vi "main.vi"() -> ()   [LabVIEW 2024]
uses:
  TypeDefs/ModeProgram.ctl
  TypeDefs/States.ctl
  TypeDefs/producent_actions.ctl
  TypeDefs/ExtendedTimer Actions.ctl
panel:
  out "Cluster":T1={"Heater1"=FALSE, "Heater2"=FALSE, "Fan"=FALSE, "MAX_TEMP"=50.0, "TEMPERATURE"=0.0, "TIMEOUT"=0.0, "Czas_do_końca"=0.0}
  out "States":T2
  in  "Plus":bool
  out "Temperature":dbl(graph)
  out "Time":string
  in  "POWER OFF":bool
  in  "Minus":bool
  in  "Start/Stop":bool
  in  "Temperature [°C]":dbl(knob) min=0.0 max=300.0 step=1.0 scale=50.0..300.0
  in  "Mode Selector":T3 scale=0.0..3.0
  # "°C"
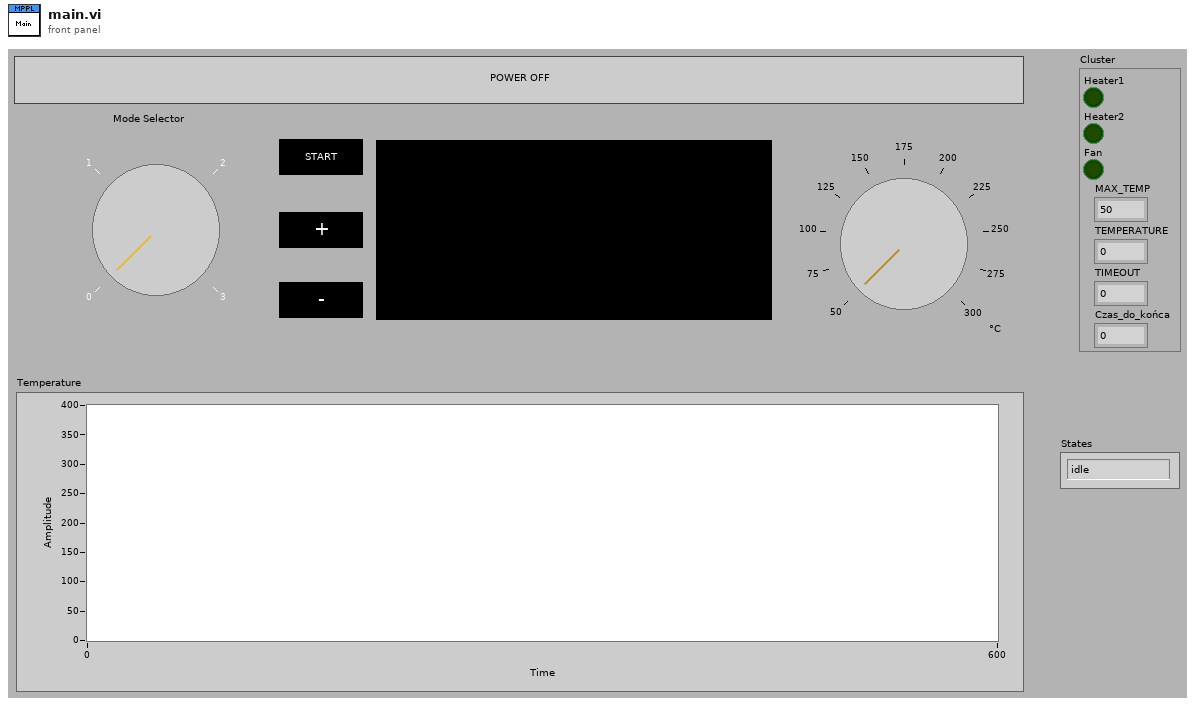
[diagram p1: front panel]
types:
  T1 = cluster{"Heater1":bool, "Heater2":bool, "Fan":bool, "MAX_TEMP":dbl, "TEMPERATURE":dbl, "TIMEOUT":dbl, "Czas_do_końca":dbl}
  T2 = typedef "States.ctl" = enum16{"idle", "reset", "heating", "stop", "exit"}
  T3 = typedef "ModeProgram.ctl" = u32
  T4 = cluster{"Heater1":bool, "Heater2":bool, "Fan":bool, "MAX_TEMP":dbl, "TEMPERATURE":dbl, "TIMEOUT":dbl, "Elapsed_Time":dbl}
  T5 = typedef "producent_actions.ctl" = enum16{"czekanie", "tryb", "temperatura", "start", "plus", "minus", "power off"}
  T6 = cluster{"Parametr":variant, "Akcje piekarnika":T5}
  T7 = typedef "ExtendedTimer Actions.ctl" = enum16{"Reset", "Check Time", "Pause", "Resume", "SetTimeOut"}
  T8 = enum8{"Enabled", "Disabled", "Disabled and Grayed Out"}
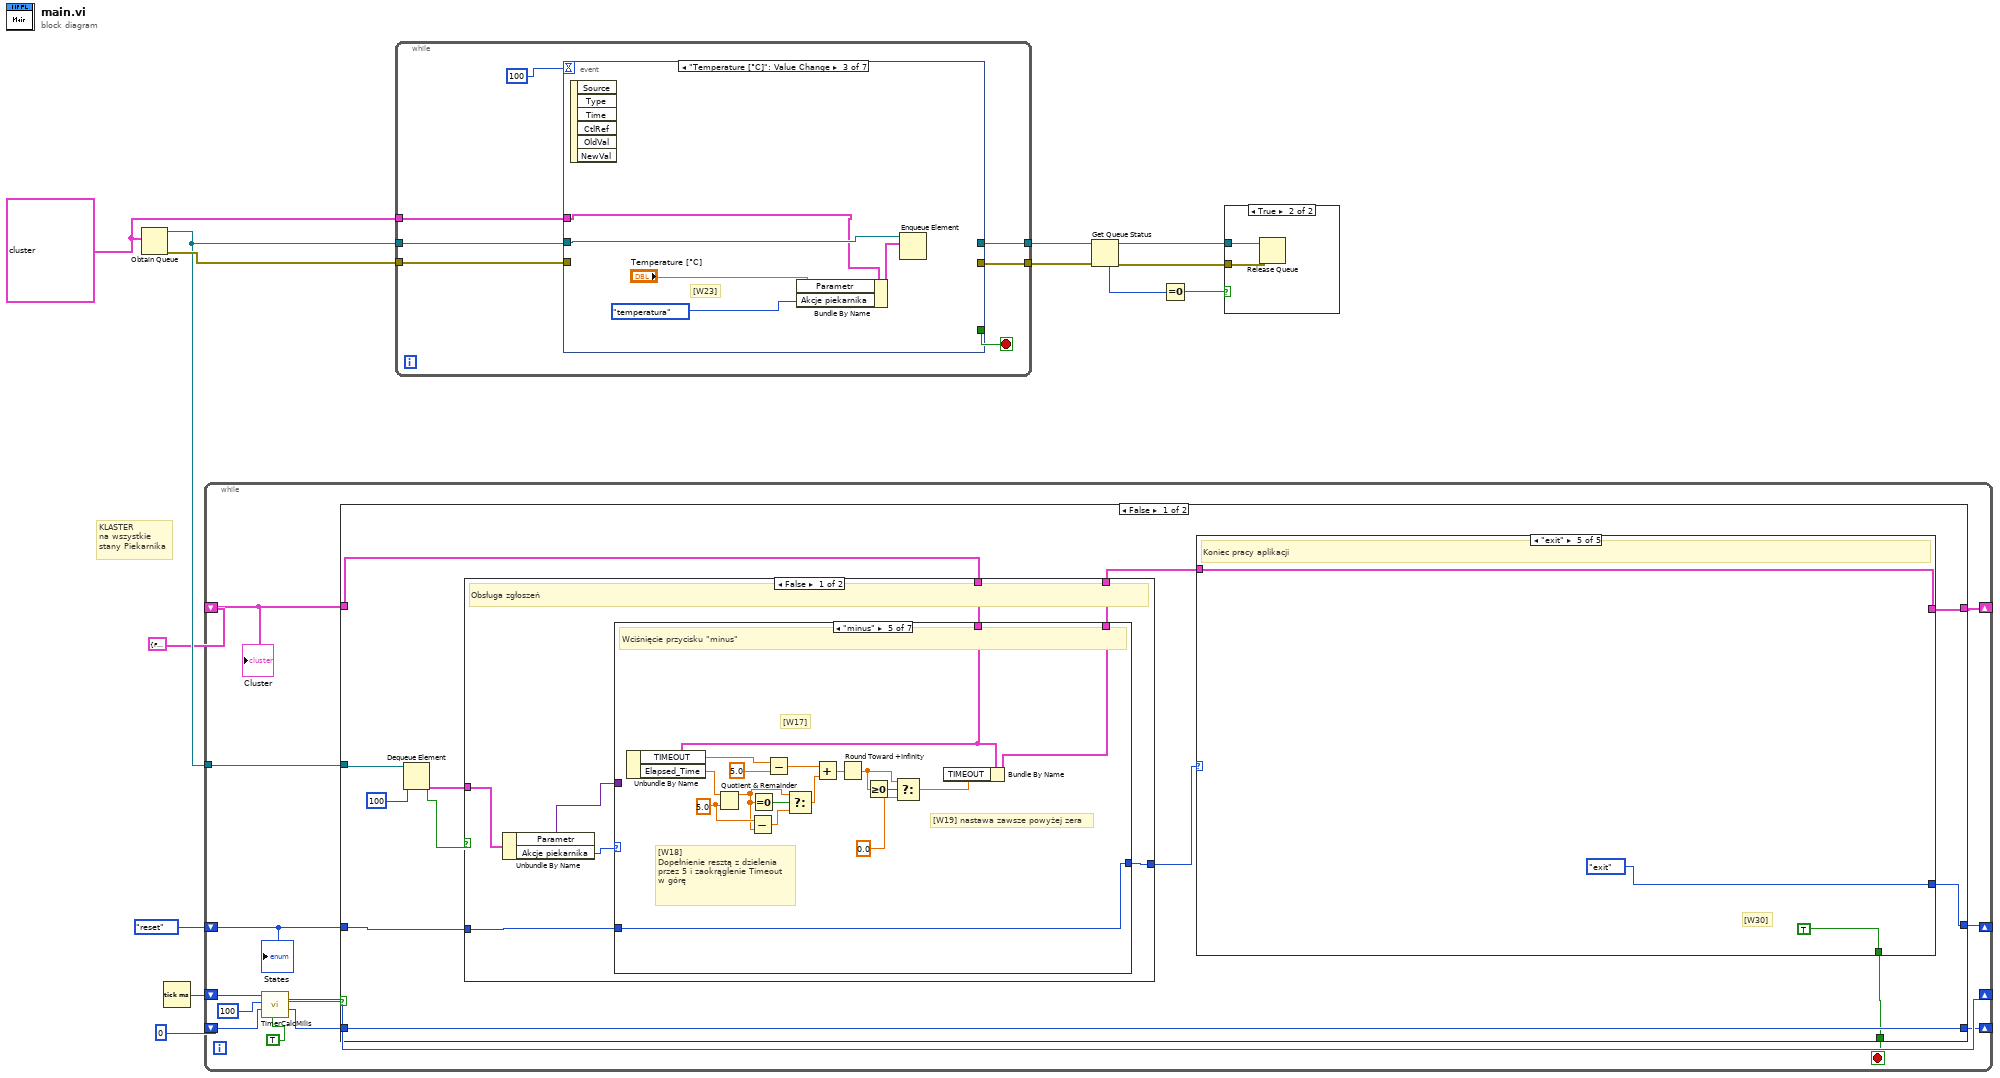
[diagram p0: block diagram]
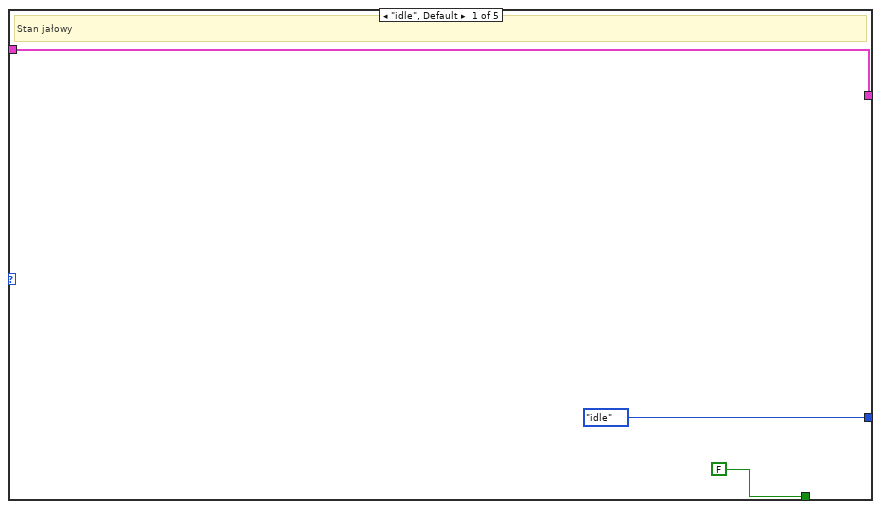
[diagram p3: hidden frame]
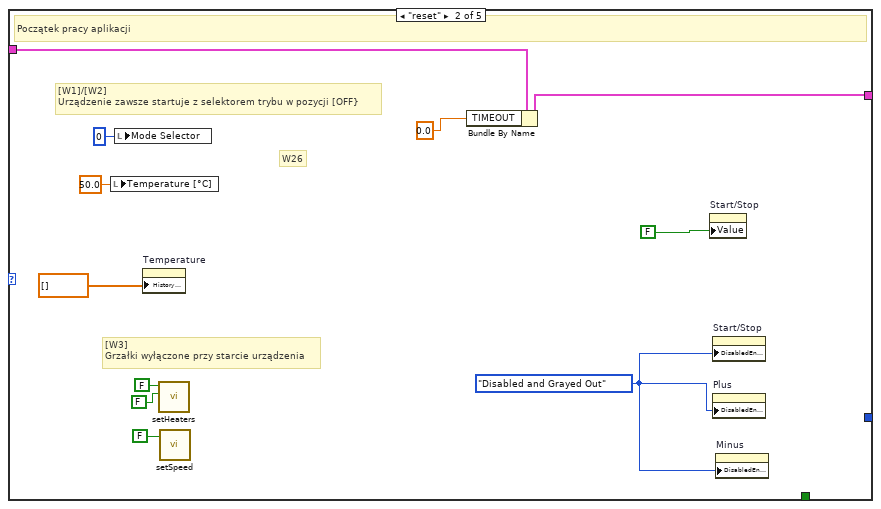
[diagram p4: hidden frame]
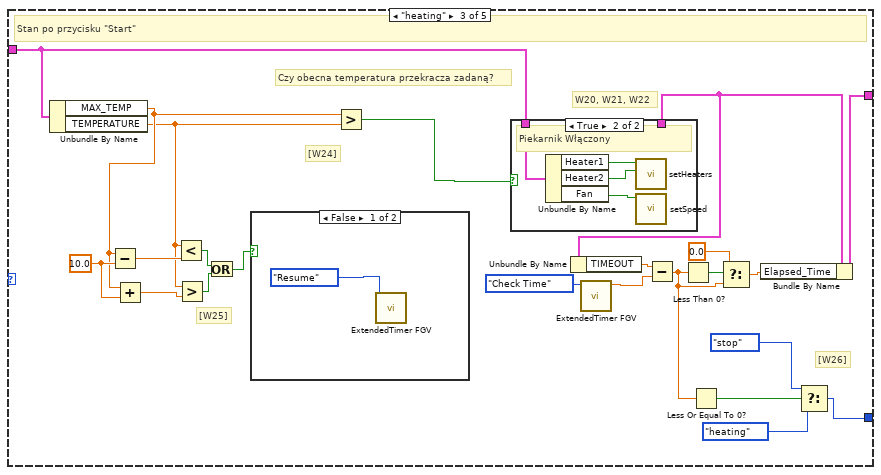
[diagram p5: hidden frame]
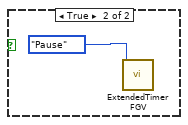
[diagram p6: hidden frame]
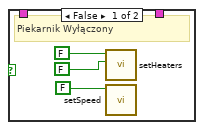
[diagram p7: hidden frame]
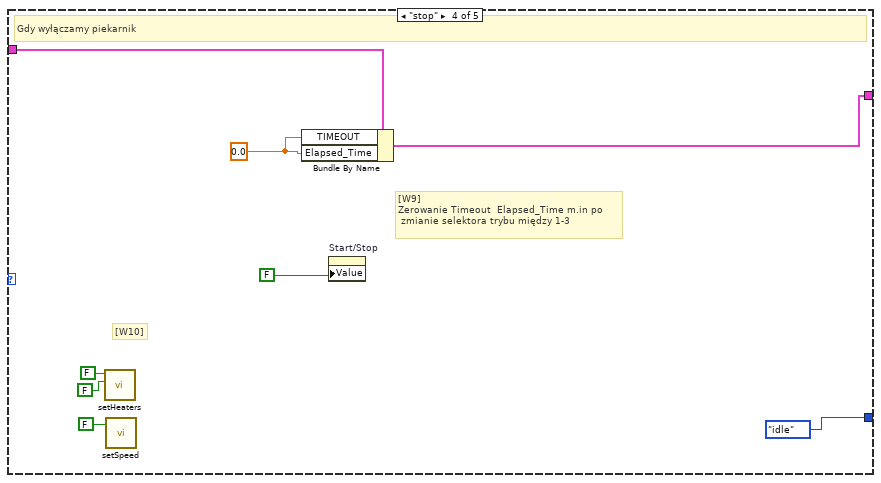
[diagram p8: hidden frame]
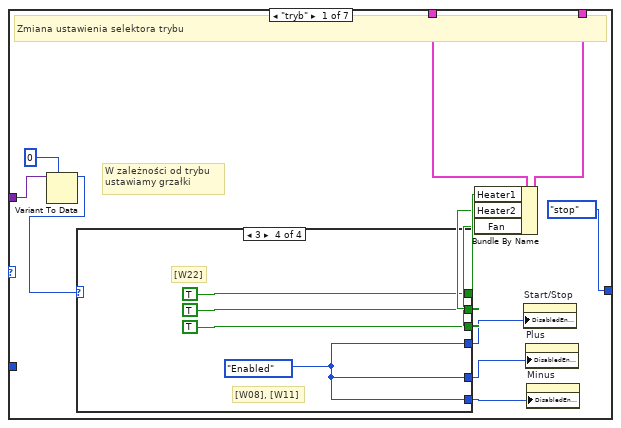
[diagram p9: hidden frame]
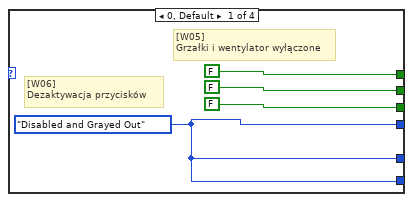
[diagram p10: hidden frame]
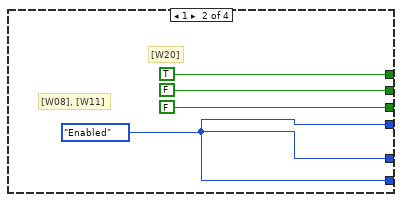
[diagram p11: hidden frame]
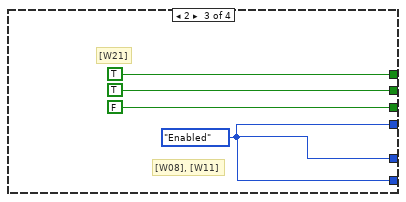
[diagram p12: hidden frame]
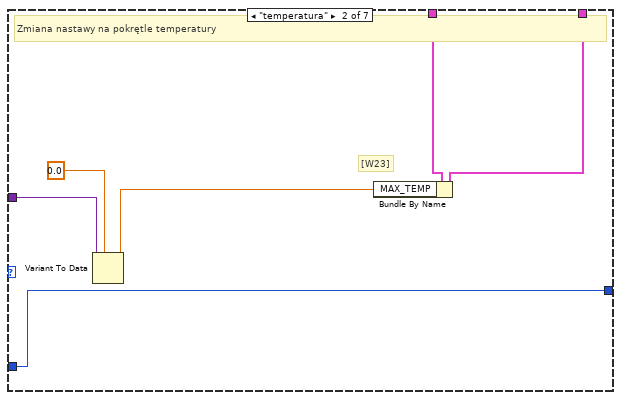
[diagram p13: hidden frame]
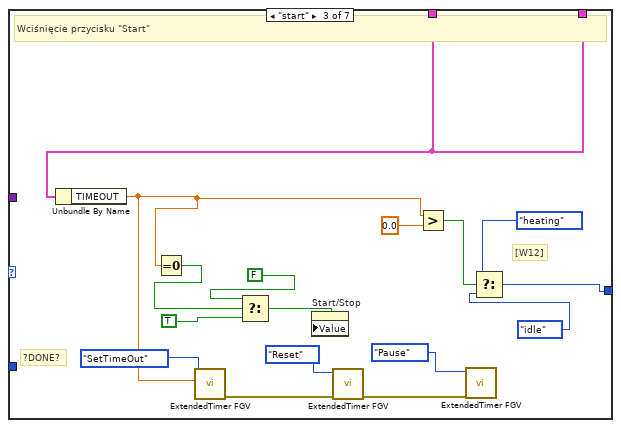
[diagram p14: hidden frame]
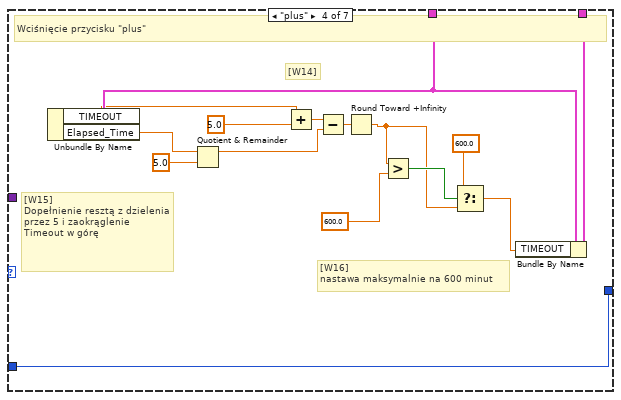
[diagram p15: hidden frame]
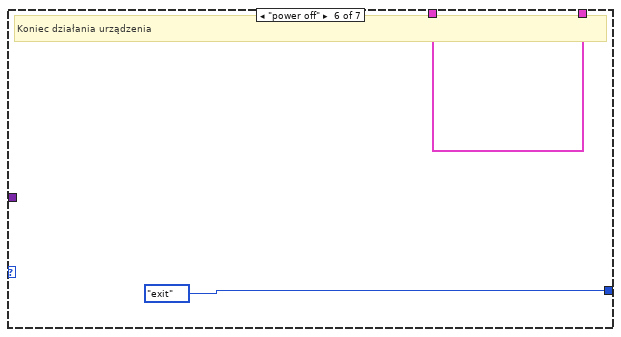
[diagram p16: hidden frame]
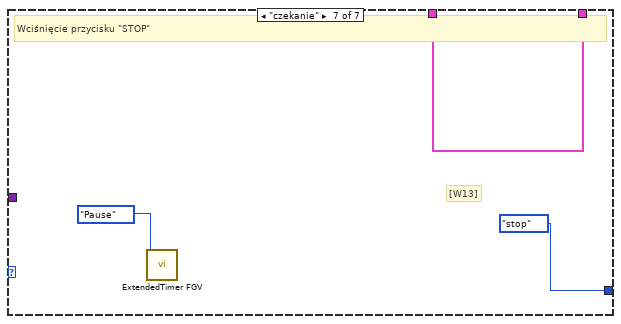
[diagram p17: hidden frame]
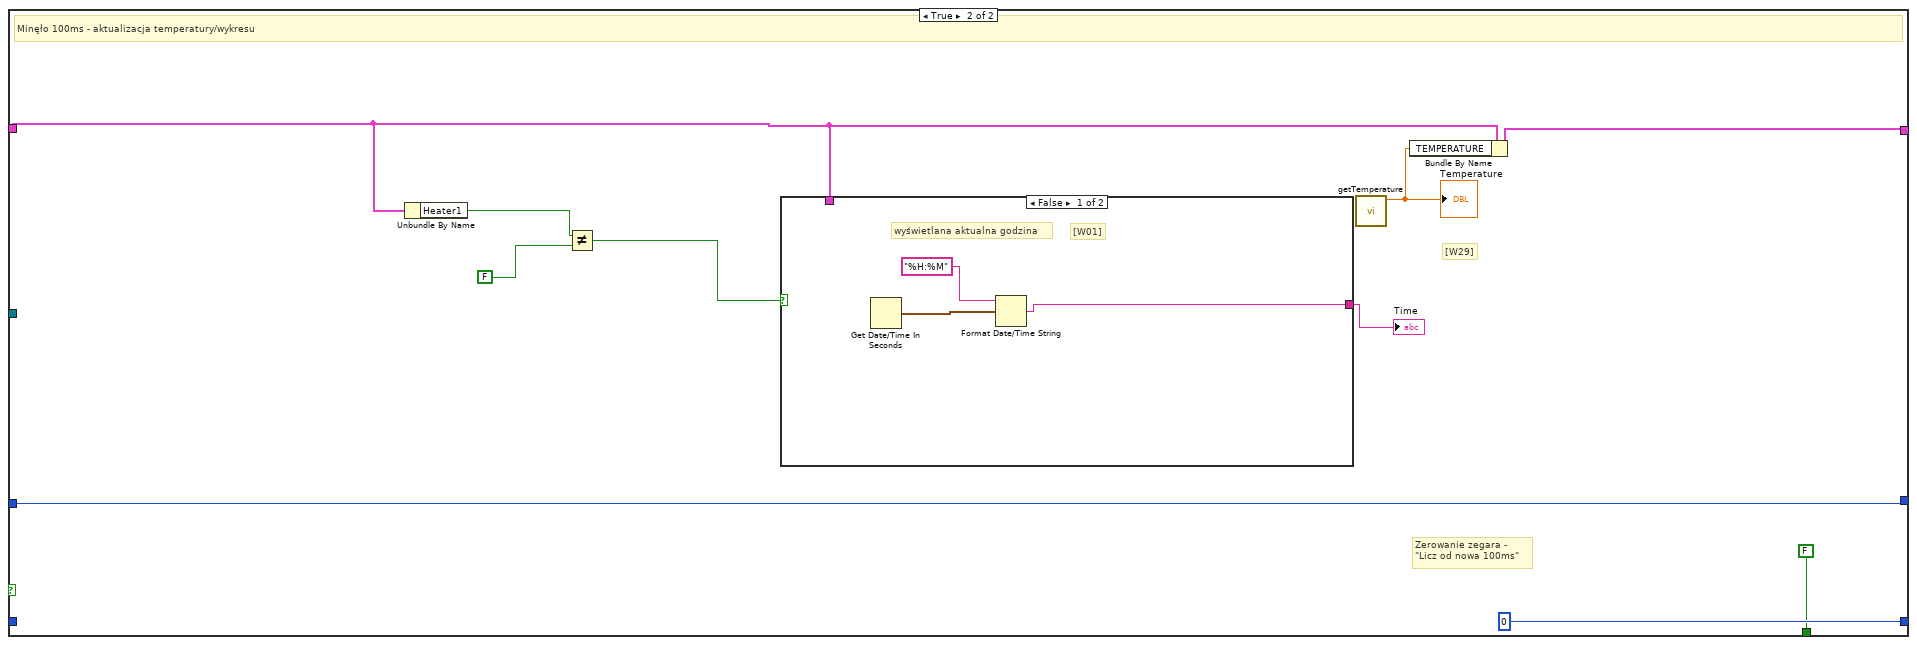
[diagram p19: hidden frame]
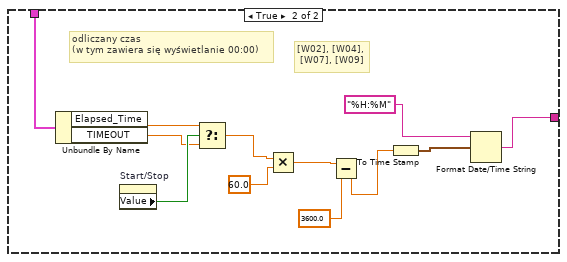
[diagram p20: hidden frame]
diagram:
  w13 = T6 {"Parametr"=variant, "Akcje piekarnika"=enum."czekanie"}
  # "KLASTER \nna wszystkie\nstany Piekarnika"
  n1 = Obtain Queue(element data type=w13) -> (queue out=w11:refnum<queue>, error out=w12:errorcluster)  [unwired: 4 in, 1 out]
  n2 = Tick Count (ms)() -> (millisecond timer value=w9:u32)
  n3 = while {
    tunnel: w11 -> [w15]
    shift-right: [w26] -> _
    shift-left: States."reset" ("States") -> [w27]
    shift-right: [w20] -> _
    shift-left: w9 -> [w23]
    shift-right: [w19] -> _
    shift-left: 0 -> [w22]
    shift-right: [w16] -> _
    shift-left: T4 {"Heater1"=FALSE, "Heater2"=FALSE, "Fan"=FALSE, "MAX_TEMP"=50.0, "TEMPERATURE"=0.0, "TIMEOUT"=0.0, "Elapsed_Time"=0.0} -> [w14]
    stop <- w17 stop-if-true
    n4 = call "TimerCalcMilis.vi"("Active"=TRUE, "ElapsedTime in"=w22, "Timeout [ms]"=u32 100, "timeOfLastCall"=w23) -> ("ElapsedTime out"=w18:u32, "Done"=w21:bool, "now"=w20:u32)  [unwired: 5 in]
    n5 = case shown="False" w21 {
      tunnel: w27 -> [w39 w199]
      tunnel: [w38 w199] -> w26
      tunnel: [w37 0] -> w19
      tunnel: w18 -> [w37 _]
      tunnel: [w36 FALSE] -> w17
      tunnel: w14 -> [w34 w198]
      tunnel: [w35 w201] -> w16
      tunnel: w15 -> [w33 _]
      frame False {
        n6 = Dequeue Element(queue=w33, timeout in ms (-1)=100) -> (element=w32:T6, timed out?=w31:bool)  [unwired: 1 in, 2 out]
        n7 = case shown="False" w31 {
          tunnel: w32 -> [w104 _]
          tunnel: w39 -> [w102 w193]
          tunnel: [w99 w193] -> w28
          tunnel: w34 -> [w101 w192]
          tunnel: [w100 w192] -> w29
          frame False {
            # "Obsługa zgłoszeń"
            n8 = Unbundle By Name(w104) -> ("Parametr"=w103:variant, "Akcje piekarnika"=w98:T5)
            n9 = case shown="\"minus\"" w98 {
              tunnel: [States."stop" ("States") w133 w148 w168 w175 States."exit" ("States") States."stop" ("States")] -> w99
              tunnel: w103 -> [w116 w138 _ _ _ _ _]
              tunnel: w102 -> [_ w133 _ w168 w175 _ _]
              tunnel: w101 -> [w105 w136 w151 w167 w185 w187 w189]
              tunnel: [w114 w135 w151 w169 w186 w187 w189] -> w100
              frame "tryb" {
                # "W zależności od trybu \nustawiamy grzałki"
                # "Zmiana ustawienia selektora trybu"
                n10 = Variant To Data(type=0, Variant=w116) -> (data=w113:i32)  [unwired: 1 in, 1 out]
                n11 = case shown="3" w113 {
                  tunnel: [FALSE TRUE TRUE TRUE] -> w112
                  tunnel: [FALSE FALSE TRUE TRUE] -> w111
                  tunnel: [FALSE FALSE FALSE TRUE] -> w110
                  tunnel: [w117 w121 w125 w129] -> w108
                  tunnel: [w117 w121 w125 w129] -> w107
                  tunnel: [w117 w121 w125 w129] -> w106
                  frame 0, Default {
                    w117 = T8."Disabled and Grayed Out" ("Disabled")
                    # "[W06]\nDezaktywacja przycisków"
                    # "[W05]\nGrzałki i wentylator wyłączone"
                  }
                  frame 1 {
                    w121 = T8."Enabled" ("Disabled")
                    # "[W20]"
                    # "[W08], [W11]"
                  }
                  frame 2 {
                    w125 = T8."Enabled" ("Disabled")
                    # "[W21]"
                    # "[W08], [W11]"
                  }
                  frame 3 {
                    w129 = T8."Enabled" ("Disabled")
                    # "[W22]"
                    # "[W08], [W11]"
                  }
                }
                n12 = Bundle By Name(cluster=w105, "Heater1"=w112, "Heater2"=w111, "Fan"=w110) -> (w114:T4)
                n13 = property on="Start/Stop" class="Bool (strict)"("DisabledEnum"=w108) -> ()  [unwired: 2 in, 2 out]
                n14 = property on="Plus" class="Bool"("DisabledEnum"=w107) -> ()  [unwired: 2 in, 2 out]
                n15 = property on="Minus" class="Bool"("DisabledEnum"=w106) -> ()  [unwired: 2 in, 2 out]
              }
              frame "temperatura" {
                # "[W23]"
                # "Zmiana nastawy na pokrętle temperatury"
                n16 = Variant To Data(type=0.0, Variant=w138) -> (data=w134:dbl)  [unwired: 1 in, 1 out]
                n17 = Bundle By Name(cluster=w136, "MAX_TEMP"=w134) -> (w135:T4)
              }
              frame "start" {
                # "[W12]"
                # "?DONE?"
                # "Wciśnięcie przycisku \"Start\""
                n18 = Unbundle By Name(w151) -> ("TIMEOUT"=w147:dbl)
                n19 = Equal To 0?(x=w147) -> (x = 0?=w146:bool)
                n20 = call "ExtendedTimer FGV.vi"("Timeout (s)"=w147, "Timer Action"=ExtendedTimer_Actions."SetTimeOut") -> ("error out"=w140:errorcluster)  [unwired: 7 in, 2 out]
                n21 = Select(t=FALSE, s=w146, f=TRUE) -> (s? t:f=w143:bool)
                n22 = property on="Start/Stop" class="Bool (strict)"("Value"=w143) -> ()  [unwired: 2 in, 2 out]
                n23 = call "ExtendedTimer FGV.vi"("error in"=w140, "Timer Action"=ExtendedTimer_Actions."Reset") -> ("error out"=w139:errorcluster)  [unwired: 7 in, 2 out]
                n24 = Greater?(x=w147, y=0.0) -> (0:w152:bool)
                n25 = call "ExtendedTimer FGV.vi"("error in"=w139, "Timer Action"=ExtendedTimer_Actions."Pause") -> ()  [unwired: 7 in, 3 out]
                n26 = Select(t=States."heating" ("States"), s=w152, f=States."idle" ("States")) -> (s? t:f=w148:T2)
              }
              frame "plus" {
                # "[W15] \nDopełnienie resztą z dzielenia przez 5 i zaokrąglenie Timeout w górę"
                # "[W16]\nnastawa maksymalnie na 600 minut"
                # "[W14]"
                # "Wciśnięcie przycisku \"plus\""
                n27 = Unbundle By Name(w167) -> ("TIMEOUT"=w166:dbl, "Elapsed_Time"=w161:dbl)
                n28 = Quotient & Remainder(x=w161, y=5.0) -> (x-y*floor(x/y)=w162:dbl)  [unwired: 1 out]
                n29 = Add(x=w166, y=5.0) -> (x+y=w164:dbl)
                n30 = Subtract(x=w164, y=w162) -> (x-y=w156:dbl)
                n31 = Round Toward +Infinity(x=w156) -> (ceil(x): smallest int >= x=w155:dbl)
                n32 = Greater?(x=w155, y=600.0) -> (0:w159:bool)
                n33 = Select(t=600.0, s=w159, f=w155) -> (s? t:f=w157:dbl)
                n34 = Bundle By Name(cluster=w167, "TIMEOUT"=w157) -> (w169:T4)
              }
              frame "minus" {
                w171 = 5.0 ("y")
                # "[W18] \nDopełnienie resztą z dzielenia przez 5 i zaokrąglenie Timeout w górę"
                # "[W17]"
                # "[W19] nastawa zawsze powyżej zera"
                # "Wciśnięcie przycisku \"minus\""
                n35 = Unbundle By Name(w185) -> ("TIMEOUT"=w183:dbl, "Elapsed_Time"=w182:dbl)
                n36 = Quotient & Remainder(x=w182, y=w171) -> (x-y*floor(x/y)=w170:dbl)  [unwired: 1 out]
                n37 = Subtract(x=w171, y=w170) -> (x-y=w172:dbl)
                n38 = Equal To 0?(x=w170) -> (x = 0?=w173:bool)
                n39 = Subtract(x=w183, y=5.0) -> (x-y=w184:dbl)
                n40 = Select(t=w170, s=w173, f=w172) -> (s? t:f=w174:dbl)
                n41 = Add(x=w184, y=w174) -> (x+y=w177:dbl)
                n42 = Round Toward +Infinity(x=w177) -> (ceil(x): smallest int >= x=w176:dbl)
                n43 = Greater Or Equal To 0?(x=w176) -> (x >= 0?=w181:bool)
                n44 = Select(t=w176, s=w181, f=0.0) -> (s? t:f=w179:dbl)
                n45 = Bundle By Name(cluster=w185, "TIMEOUT"=w179) -> (w186:T4)
              }
              frame "power off" {
                # "Koniec działania urządzenia"
              }
              frame "czekanie" {
                # "[W13]"
                # "Wciśnięcie przycisku \"STOP\""
                n46 = call "ExtendedTimer FGV.vi"("Timer Action"=ExtendedTimer_Actions."Pause") -> ()  [unwired: 8 in, 3 out]
              }
            }
          }
          frame True {
            # "Przy IDLE/Heating wystarczy\nPuścić dalej zapętlony stan\nz poprzedniej iteracji"
            # "Brak zgłoszeń/ lub błąd  = IDLE lub inny z poprzedniej iteracji"
          }
        }
        n47 = case shown="\"exit\"" w28 {
          tunnel: [States."idle" ("States") _ w70 States."idle" ("States") States."exit" ("States")] -> w38
          tunnel: [FALSE _ _ _ TRUE] -> w36
          tunnel: [w40 w49 w75 w89 w95] -> w35
          tunnel: w29 -> [w40 w50 w76 w91 w95]
          frame "idle", Default {
            # "Stan jałowy"
          }
          frame "reset" {
            w45 = T8."Disabled and Grayed Out" ("Disabled")
            # "[W3]\nGrzałki wyłączone przy starcie urządzenia"
            # "[W1]/[W2]\nUrządzenie zawsze startuje z selektorem trybu w pozycji [OFF}"
            # "W26"
            # "Początek pracy aplikacji"
            n48 = local write "Temperature [°C]"(50.0 ("Temperature [°C]")) -> ()
            n49 = local write "Mode Selector"(T3 0 ("Mode Selector")) -> ()
            n50 = property on="Temperature" class="WFChart (strict)"("History Data"=dbl[] []) -> ()  [unwired: 2 in, 2 out]
            n51 = call "setHeaters.vi"("Heater2"=FALSE ("Heater1"), "Heater1"=FALSE) -> ()  [unwired: 9 in, 1 out]
            n52 = call "setSpeed.vi"("Speed"=FALSE ("Heater1")) -> ()  [unwired: 10 in, 1 out]
            n53 = Bundle By Name(cluster=w50, "TIMEOUT"=0.0) -> (w49:T4)
            n54 = property on="Start/Stop" class="Bool (strict)"("Value"=FALSE) -> ()  [unwired: 2 in, 2 out]
            n55 = property on="Start/Stop" class="Bool (strict)"("DisabledEnum"=w45) -> ()  [unwired: 2 in, 2 out]
            n56 = property on="Plus" class="Bool"("DisabledEnum"=w45) -> ()  [unwired: 2 in, 2 out]
            n57 = property on="Minus" class="Bool"("DisabledEnum"=w45) -> ()  [unwired: 2 in, 2 out]
          }
          frame "heating" {
            w60 = 10.0 ("y")
            # "[W25]"
            # "[W26]"
            # "[W24]"
            # "W20, W21, W22"
            # "Czy obecna temperatura przekracza zadaną?"
            # "Stan po przycisku \"Start\""
            n58 = Unbundle By Name(w76) -> ("MAX_TEMP"=w59:dbl, "TEMPERATURE"=w58:dbl)
            n59 = Subtract(x=w59, y=w60) -> (x-y=w68:dbl)
            n60 = Add(x=w59, y=w60) -> (x+y=w57:dbl)
            n61 = Less?(x=w58, y=w68) -> (x < y?=w56:bool)
            n62 = Greater?(x=w58, y=w57) -> (0:w55:bool)
            n63 = Or(x=w56, y=w55) -> (x .or. y?=w54:bool)
            n64 = case shown="False" w54 {
              frame False {
                n65 = call "ExtendedTimer FGV.vi"("Timer Action"=ExtendedTimer_Actions."Resume") -> ()  [unwired: 8 in, 3 out]
              }
              frame True {
                n66 = call "ExtendedTimer FGV.vi"("Timer Action"=ExtendedTimer_Actions."Pause") -> ()  [unwired: 8 in, 3 out]
              }
            }
            n67 = Greater?(x=w59, y=w58) -> (0:w65:bool)
            n68 = case shown="True" w65 {
              tunnel: w76 -> [w82 w86]
              tunnel: [w82 w86] -> w74
              frame False {
                # "Piekarnik Wyłączony"
                n69 = call "setHeaters.vi"("Heater2"=FALSE, "Heater1"=FALSE) -> ()  [unwired: 9 in, 1 out]
                n70 = call "setSpeed.vi"("Speed"=FALSE) -> ()  [unwired: 10 in, 1 out]
              }
              frame True {
                # "Piekarnik Włączony"
                n71 = Unbundle By Name(w86) -> ("Heater1"=w85:bool, "Heater2"=w84:bool, "Fan"=w83:bool)
                n72 = call "setHeaters.vi"("Heater2"=w84, "Heater1"=w85) -> ()  [unwired: 9 in, 1 out]
                n73 = call "setSpeed.vi"("Speed"=w83) -> ()  [unwired: 10 in, 1 out]
              }
            }
            n74 = Unbundle By Name(w74) -> ("TIMEOUT"=w73:dbl)
            n75 = call "ExtendedTimer FGV.vi"("Timer Action"=ExtendedTimer_Actions."Check Time") -> ("Elapsed Time"=w67:dbl)  [unwired: 8 in, 2 out]
            n76 = Subtract(x=w73, y=w67) -> (x-y=w63:dbl)
            n77 = Less Than 0?(x=w63) -> (x < 0?=w64:bool)
            n78 = Less Or Equal To 0?(x=w63) -> (x <= 0?=w66:bool)
            n79 = Select(t=0.0, s=w64, f=w63) -> (s? t:f=w61:dbl)
            n80 = Bundle By Name(cluster=w74, "Elapsed_Time"=w61) -> (w75:T4)
            n81 = Select(t=States."stop" ("States"), s=w66, f=States."heating" ("States")) -> (s? t:f=w70:T2)
          }
          frame "stop" {
            w90 = 0.0
            # "[W9] \nZerowanie Timeout  Elapsed_Time m.in po \n zmianie selektora trybu między 1-3"
            # "[W10]"
            # "Gdy wyłączamy piekarnik"
            n82 = call "setHeaters.vi"("Heater2"=FALSE ("Heater1"), "Heater1"=FALSE) -> ()  [unwired: 9 in, 1 out]
            n83 = call "setSpeed.vi"("Speed"=FALSE ("Heater1")) -> ()  [unwired: 10 in, 1 out]
            n84 = Bundle By Name(cluster=w91, "TIMEOUT"=w90, "Elapsed_Time"=w90) -> (w89:T4)
            n85 = property on="Start/Stop" class="Bool (strict)"("Value"=FALSE) -> ()  [unwired: 2 in, 2 out]
          }
          frame "exit" {
            # "[W30]"
            # "Koniec pracy aplikacji"
          }
        }
      }
      frame True {
        # "Zerowanie zegara -\n\"Licz od nowa 100ms\""
        # "[W29]"
        # "Minęło 100ms - aktualizacja temperatury/wykresu"
        n86 = Unbundle By Name(w198) -> ("Heater1"=w196:bool)
        n87 = Not Equal?(x=w196, y=FALSE) -> (x != y?=w195:bool)
        n88 = case shown="False" w195 {
          tunnel: [w204 w212] -> w194
          tunnel: w198 -> [_ w215]
          frame False {
            # "[W01]"
            # "wyświetlana aktualna godzina"
            n89 = Get Date/Time In Seconds() -> (seconds since 1Jan1904=w206:timestamp)
            n90 = Format Date/Time String(time format string (%c)="%H:%M", seconds (now)=w206) -> (date/time string=w204:string)  [unwired: 1 in]
          }
          frame True {
            # "[W02], [W04],\n [W07], [W09]"
            # "odliczany czas \n(w tym zawiera się wyświetlanie 00:00)"
            n91 = Unbundle By Name(w215) -> ("Elapsed_Time"=w216:dbl, "TIMEOUT"=w217:dbl)
            n92 = property on="Start/Stop" class="Bool (strict)"() -> ("Value"=w218:bool)  [unwired: 2 in, 2 out]
            n93 = Select(t=w216, s=w218, f=w217) -> (s? t:f=w211:dbl)
            n94 = Multiply(x=w211, y=60.0) -> (x*y=w209:dbl)
            n95 = Subtract(x=w209, y=3600.0) -> (x-y=w208:dbl)
            n96 = To Time Stamp(1:w208) -> (0:w213:timestamp)
            n97 = Format Date/Time String(time format string (%c)="%H:%M", seconds (now)=w213) -> (date/time string=w212:string)  [unwired: 1 in]
          }
        }
        "Time" <- w194
        n98 = call "getTemperature.vi"() -> ("Temperature"=w200:dbl)  [unwired: 10 in, 1 out]
        "Temperature" <- w200
        n99 = Bundle By Name(cluster=w198, "TEMPERATURE"=w200) -> (w201:T4)
      }
    }
    "States" <- w27
    "Cluster" <- w14
  }
  n100 = while {
    tunnel: w11 -> [w223]
    tunnel: w13 -> [w222]
    tunnel: w12 -> [w221]
    tunnel: [w220] -> w6
    tunnel: [w219] -> w5
    stop <- w224 stop-if-true
    n101 = event shown="[2] \"Temperature [°C]\": Value Change" {
      selector: _ -> [_ _ _ _ _ _ _]
      dyn-events: _ -> [_ _ _ _ _ _ _]
      timeout: 100 -> [_ _ _ _ _ _ _]
      tunnel: [_ _ _ _ _ _ "POWER OFF"] -> w224
      tunnel: w223 -> [_ w230 w235 w238 w241 w249 w255]
      tunnel: w222 -> [_ w229 w234 w237 w242 w248 w256]
      tunnel: w221 -> [_ _ _ _ _ _ w254]
      tunnel: [_ _ _ _ _ _ w253] -> w220
      tunnel: [_ _ _ _ _ _ w252] -> w219
      event Timeout {
        n102 = event-data() -> ()  [unwired: 1 in, 3 out]
      }
      event Value Change {
        n103 = event-data() -> ()  [unwired: 1 in, 6 out]
        n104 = Bundle By Name(cluster=w229, "Parametr"="Mode Selector", "Akcje piekarnika"=producent_actions."tryb") -> (w227:T6)
        n105 = Enqueue Element(queue=w230, element=w227) -> ()  [unwired: 2 in, 3 out]
      }
      event "Temperature [°C]": Value Change {
        # "[W23]"
        n106 = event-data() -> ()  [unwired: 1 in, 6 out]
        n107 = Bundle By Name(cluster=w234, "Parametr"="Temperature [°C]", "Akcje piekarnika"=producent_actions."temperatura") -> (w233:T6)
        n108 = Enqueue Element(queue=w235, element=w233) -> ()  [unwired: 2 in, 3 out]
      }
      event "Plus": Value Change {
        n109 = event-data() -> ()  [unwired: 1 in, 6 out]
        n110 = Bundle By Name(cluster=w237, "Akcje piekarnika"=producent_actions."plus") -> (w239:T6)
        n111 = Enqueue Element(queue=w238, element=w239) -> ()  [unwired: 2 in, 3 out]
      }
      event "Minus": Value Change {
        n112 = event-data() -> ()  [unwired: 1 in, 6 out]
        n113 = Bundle By Name(cluster=w242, "Akcje piekarnika"=producent_actions."minus" ("Akcje piekarnika 2")) -> (w243:T6)
        n114 = Enqueue Element(queue=w241, element=w243) -> ()  [unwired: 2 in, 3 out]
      }
      event "Start/Stop": Value Change {
        n115 = event-data() -> ()  [unwired: 1 in, 6 out]
        n116 = Select(t=producent_actions."start" ("Akcje piekarnika 2"), s="Start/Stop", f=producent_actions."czekanie" ("Akcje piekarnika 2")) -> (s? t:f=w246:T5)
        n117 = Bundle By Name(cluster=w248, "Akcje piekarnika"=w246) -> (w247:T6)
        n118 = Enqueue Element(queue=w249, element=w247) -> ()  [unwired: 2 in, 3 out]
      }
      event "POWER OFF": Value Change {
        # "[W30]"
        n119 = event-data() -> ()  [unwired: 1 in, 6 out]
        n120 = Bundle By Name(cluster=w256, "Akcje piekarnika"=producent_actions."power off") -> (w257:T6)
        n121 = Enqueue Element(queue=w255, element=w257, error in (no error)=w254) -> (queue out=w253:refnum<queue>, error out=w252:errorcluster)  [unwired: 1 in, 1 out]
      }
    }
  }
  n122 = Get Queue Status(queue=w6, error in (no error)=w5) -> (queue out=w2:refnum<queue>, error out=w1:errorcluster, # elements in queue=w4:i32)  [unwired: 1 in, 5 out]
  n123 = Equal To 0?(x=w4) -> (x = 0?=w3:bool)
  n124 = case shown="True" w3 {
    tunnel: w2 -> [_ w260]
    tunnel: w1 -> [_ w259]
    frame False {
    }
    frame True {
      n125 = Release Queue(queue=w260, error in (no error)=w259) -> ()  [unwired: 1 in, 3 out]
    }
  }
